vi "init.vi"(8 "error in (no error)":errorcluster, 11 "EncoderReaderTC in":refnum<class "EncoderReaderTC.lvclass">) -> (0 "error out":errorcluster, 3 "EncoderReaderTC out":refnum<class "EncoderReaderTC.lvclass">)   [LabVIEW 2013, in "EncoderReaderTC.lvclass"]
uses:
  EncoderReaderTC.lvclass
  <userlib>/Common/Devices/EncoderReader/Config/Encoder Reader.ctl
  <userlib>/Common/SerialProtocols/Configuration/SerialConfig.ctl
  <userlib>/Common/SerialProtocols/Configuration/SerialProtocol.ctl
  <userlib>/Common/SerialProtocols/Configuration/ProtocolParameters.ctl
  <userlib>/Common/SerialProtocols/Configuration/SerialMessageParameters.ctl
  <userlib>/Common/Devices/EncoderReader/EncoderReader/EncoderReader.lvclass/EncoderReader.ctl
  <userlib>/Common/Devices/EncoderReader/EncoderReader/EncoderReader.lvclass
  ConfigurationThisComponent/ConfigurationThisComponent.lvclass
  <userlib>/Common/SerialProtocols/SerialProtocols.lvlib
  <userlib>/Common/Devices/EncoderReader/EncoderReader.lvlib
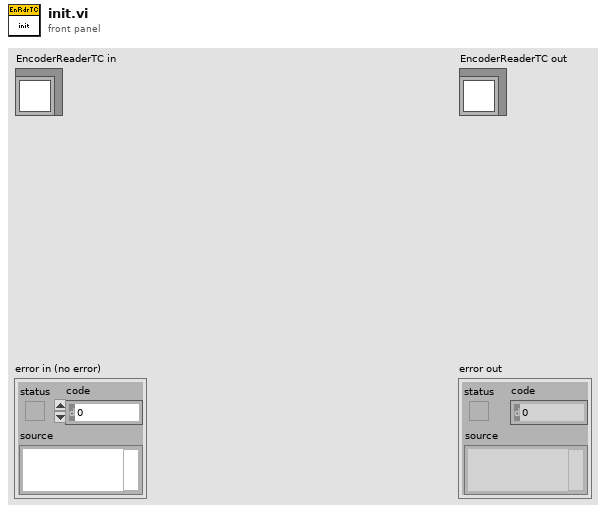
[diagram p1: front panel]
types:
  T1 = typedef "EncoderReader.lvlib/Encoder Reader.ctl" = cluster{"Serial":T2}
  T2 = typedef "SerialProtocols.lvlib/SerialConfig.ctl" = cluster{"Serial Protocol":T3, "Protocol Parameters":T4, "Serial Message Parameters":T5}
  T3 = typedef "SerialProtocols.lvlib/SerialProtocol.ctl" = enum16{"RS232", "RS485", "SerialSimulator"}
  T4 = typedef "SerialProtocols.lvlib/ProtocolParameters.ctl" = cluster{"VISA resource name":refnum<visa-resource-name>, "Baud Rate":u32, "Data Bits":u16, "Parity":enum16{"None", "Odd", "Even", "Mark", "Space"}, "Flow Control":u16, "Stop Bits":u16, "Timeout (ms)":u32}
  T5 = typedef "SerialProtocols.lvlib/SerialMessageParameters.ctl" = cluster{"Byte Count":u32, "Enable Termination Character":bool, "Termination Char":u8}
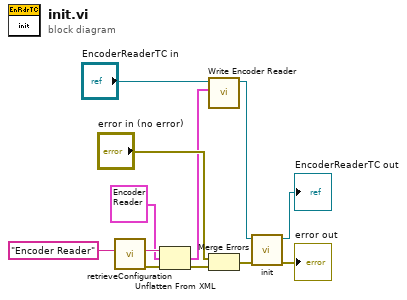
[diagram p0: block diagram]
diagram:
  n1 = call "retrieveConfiguration.vi"("configName"="Encoder Reader") -> ("error out"=w8:errorcluster, "xmlConfig"=w9:string)  [unwired: 8 in, 1 out]
  n2 = Unflatten From XML(xml string=w9, type=T1 {"Serial"={"Serial Protocol"=enum."RS485", "Protocol Parameters"={"VISA resource name"="", "Baud Rate"=9600, "Data Bits"=8, "Parity"=enum."None", "Flow Control"=0, "Stop Bits"=10, "Timeout (ms)"=10000}, "Serial Message Parameters"={"Byte Count"=200, "Enable Termination Character"=FALSE, "Termination Char"=200}}} ("Encoder Reader"), error in (no error)=w8) -> (value=w1:T1, error out=w5:errorcluster)
  n3 = call <userlib>:"Write Encoder Reader.vi"("Encoder Reader"=w1, "EncoderReader in"="EncoderReaderTC in") -> ("EncoderReader out"=w2:refnum<class "EncoderReaderTC.lvclass">)  [unwired: 9 in]
  n4 = Merge Errors("error in (no error)", w5) -> (w4:errorcluster)
  n5 = call-parent "init.vi"("error in (no error)"=w4, "EncoderReader in"=w2) -> ("error out"=→"error out":errorcluster, "EncoderReader out"=→"EncoderReaderTC out":refnum<class "EncoderReaderTC.lvclass">)  [unwired: 8 in]
